vi "Is a textual Guardian.vi"(8 "error in (no error)":errorcluster, 10 "Target GD ID":string) -> (0 "error out":errorcluster, 2 "Textual?":bool)   [LabVIEW 2026, in "TALOS.lvlib"]
uses:
  TALOS.lvlib
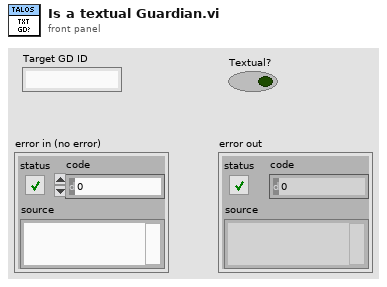
[diagram p1: front panel]
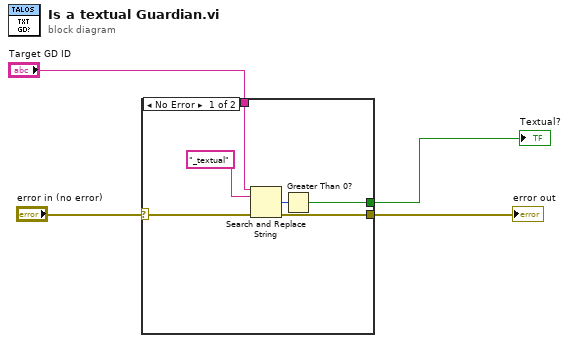
[diagram p0: block diagram]
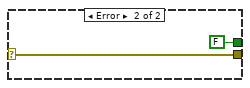
[diagram p2: hidden frame]
diagram:
  n1 = case shown="No Error" "error in (no error)" {
    selector: "error in (no error)" -> [w5 w12]
    tunnel: "Target GD ID" -> [w10 _]
    tunnel: [w9 FALSE] -> w3
    tunnel: [w6 w12] -> w2
    frame No Error {
      n2 = Search and Replace String(input string=w10, search string="_textual", error in=w5) -> (number of replacements=w8:i32, error out=w6:errorcluster)  [unwired: 5 in, 2 out]
      n3 = Greater Than 0?(x=w8) -> (x > 0?=w9:bool)
    }
    frame Error {
    }
  }
  "Textual?" <- w3
  "error out" <- w2
